vi "ADO Connection Open.vi"(6 "Password":string, 7 "UserID":string, 8 "error in (no error)":errorcluster, 10 "ConnectionString":string, 11 "ADODB._Connection In":refnum<k7>) -> (0 "error out":errorcluster, 3 "ADODB._Connection Out":refnum<k7>)   [LabVIEW 2014]
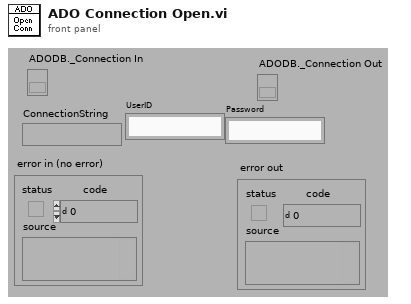
[diagram p1: front panel]
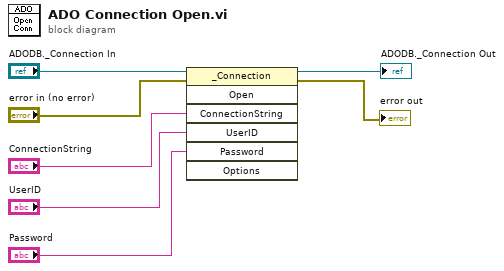
[diagram p0: block diagram]
diagram:
  n1 = invoke class="_Connection" method="Open"(reference="ADODB._Connection In", error in="error in (no error)", "ConnectionString"="ConnectionString", "UserID"="UserID", "Password"="Password") -> (reference out=→"ADODB._Connection Out":refnum<k7>, error out=→"error out":errorcluster)  [unwired: 2 in, 5 out]
